vi "Add.vi"(7 "Top Level Library?":bool, 8 "error in (no error)":errorcluster, 10 "ProjectItem Refnum":refnum<vi>, 11 "PPL in":refnum<class "NI_AB_API_PPL.lvclass">) -> (0 "error out":errorcluster, 3 "PPL out":refnum<class "NI_AB_API_PPL.lvclass">)   [LabVIEW 2020, in "NI_AB_API_PPL.lvclass"]
uses:
  <vilib>/AppBuilder/AB_API/PPL/NI_AB_API_PPL.lvclass
  e:/builds/penguin/labview/branches/2020/dev/dist/vi.lib/AppBuilder/AB_API/Build/NI_AB_API_Build.lvclass
  <vilib>/AppBuilder/AB_Classes/PackedLib/AB_PackedLibrary.lvclass
  e:/builds/penguin/labview/branches/2020/dev/dist/vi.lib/AppBuilder/AB_Classes/Build/AB_Build.lvclass
  <vilib>/AppBuilder/AB_API/PPL/NI_AB_API_PPL.lvclass/NI_AB_API_PPL.ctl
  <vilib>/AppBuilder/AB_Classes/Build/AB_Build.lvclass
  <vilib>/AppBuilder/AB_Classes/Source/AB_Source.lvclass
  <vilib>/AppBuilder/AB_API/Build/NI_AB_API_Build.lvclass
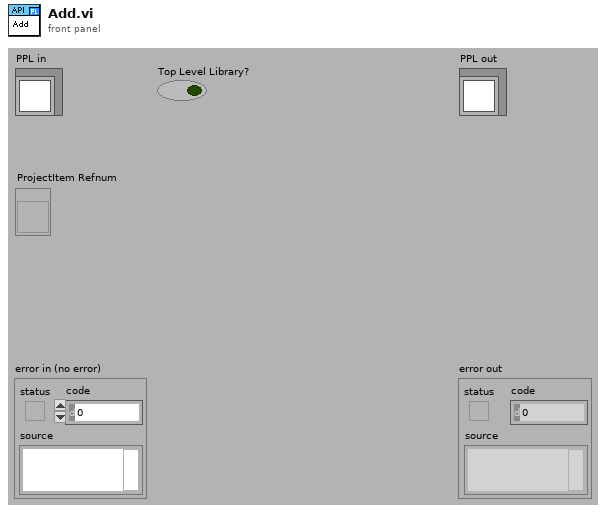
[diagram p1: front panel]
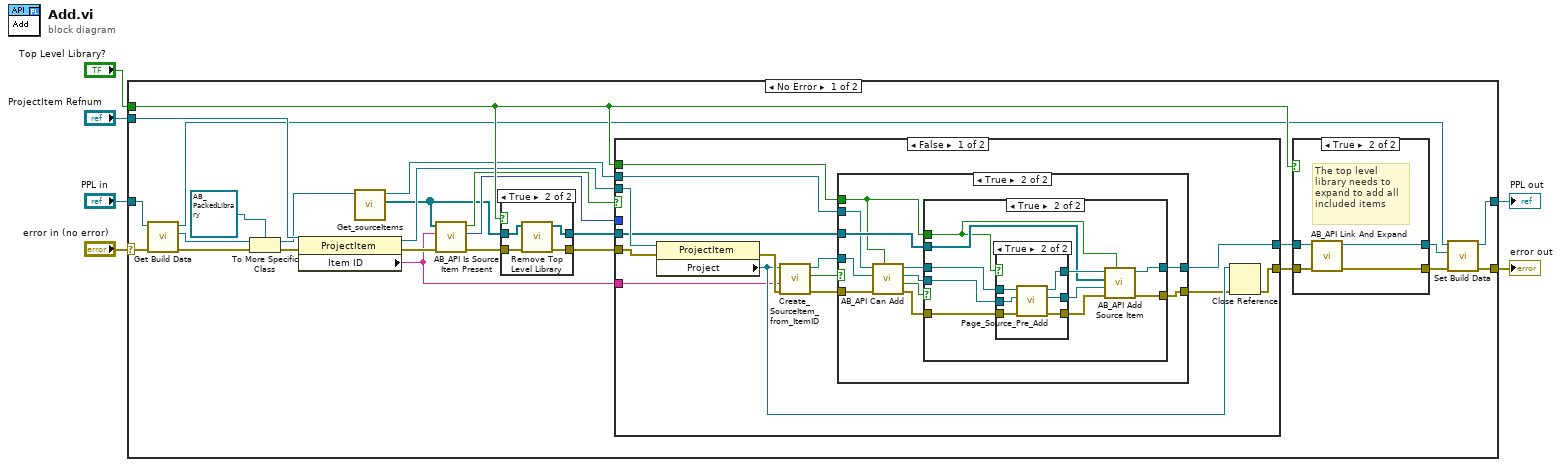
[diagram p0: block diagram]
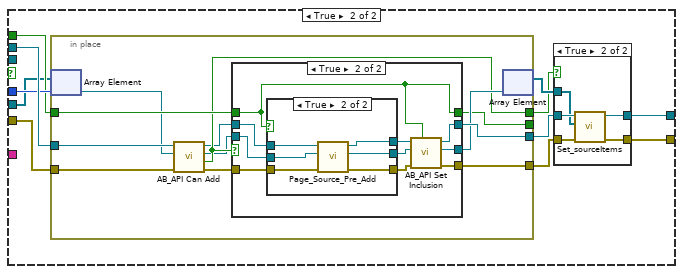
[diagram p7: hidden frame]
diagram:
  n1 = case shown="No Error" "error in (no error)" {
    selector: "error in (no error)" -> [w31 w147]
    tunnel: [w11 w147] -> w5
    tunnel: [w13 w146] -> w3
    tunnel: "PPL in" -> [w8 w146]
    tunnel: "ProjectItem Refnum" -> [w32 _]
    tunnel: "Top Level Library?" -> [w30 _]
    frame No Error {
      n2 = call <vilib>:"Get Build Data.vi"("error in (no error)"=w31, "NI_AB_API_Build in"=w8) -> ("error out"=w16:errorcluster, "AB_Build.lvclass"=w9:refnum<class "AB_Build.lvclass">, "NI_AB_API_Build out"=w7:refnum<class "NI_AB_API_PPL.lvclass">)  [unwired: 7 in]
      n3 = To More Specific Class(target class=refnum<class "AB_PackedLibrary.lvclass"> refnum ("AB_PackedLibrary.lvclass"), reference=w9, error in=w16) -> (specific class reference=w14:refnum<class "AB_PackedLibrary.lvclass">, error out=w15:errorcluster)
      n4 = property class="ProjectItem"(reference=w32, error in=w15) -> (reference out=w29:refnum<vi>, error out=w26:errorcluster, "Item ID"=w25:string)
      n5 = call <vilib>:"Get_sourceItems.vi"("Class in"=w14) -> ("sourceItems"=w23:refnum<class "AB_Source.lvclass">[], "Class out"=w28:refnum<class "AB_PackedLibrary.lvclass">)  [unwired: 8 in, 1 out]
      n6 = call <vilib>:"AB_API Is Source Item Present.vi"("error in"=w26, "item ID"=w25, "source items"=w23) -> ("error out"=w21:errorcluster, "index"=w24:i32, "source item present?"=w27:bool)  [unwired: 6 in]
      n7 = case shown="True" w30 {
        tunnel: w23 -> [w40 w44]
        tunnel: [w40 w43] -> w22
        tunnel: w21 -> [w39 w42]
        tunnel: [w39 w41] -> w20
        frame False {
        }
        frame True {
          n8 = call <vilib>:"Remove Top Level Library.vi"("error in"=w42, "sourceItems"=w44) -> ("error out"=w41:errorcluster, "sourceItems out"=w43:refnum<class "AB_Source.lvclass">[])  [unwired: 7 in]
        }
      }
      n9 = case shown="False" w27 {
        tunnel: w29 -> [w58 _]
        tunnel: [w54 w100] -> w19
        tunnel: [w50 w98] -> w18
        tunnel: w20 -> [w49 w94]
        tunnel: w28 -> [w48 w103]
        tunnel: w25 -> [w47 _]
        tunnel: w22 -> [w46 w95]
        tunnel: w24 -> [_ w102]
        tunnel: w30 -> [w45 w97]
        frame False {
          n10 = property class="ProjectItem"(reference=w58, error in=w49) -> (error out=w57:errorcluster, "Project"=w52:refnum<vi>)  [unwired: 1 out]
          n11 = call <vilib>:"Create_SourceItem_from_ItemID.vi"("error in (no error)"=w57, "itemID"=w47, "Project Refnum"=w52) -> ("error out"=w55:errorcluster, "valid?"=w53:bool, "AB_Source out"=w56:refnum<class "AB_Source.lvclass">)  [unwired: 6 in]
          n12 = case shown="True" w53 {
            tunnel: w56 -> [_ w68]
            tunnel: w55 -> [w59 w64]
            tunnel: w48 -> [w60 w67]
            tunnel: [w60 w71] -> w54
            tunnel: [w59 w70] -> w51
            tunnel: w46 -> [_ w69]
            tunnel: w45 -> [_ w61]
            frame False {
            }
            frame True {
              n13 = call <vilib>:"AB_API Can Add.vi"("top tree? (true)"=w61, "error in (no error)"=w64, "AB_Source in"=w68, "Build in"=w67) -> ("error out"=w63:errorcluster, "can add?"=w62:bool, "AB_Source out"=w65:refnum<class "AB_Source.lvclass">, "Build out"=w66:refnum<class "AB_PackedLibrary.lvclass">)  [unwired: 4 in]
              n14 = case shown="True" w62 {
                tunnel: w66 -> [w73 w81]
                tunnel: [w73 w82] -> w71
                tunnel: [w72 w83] -> w70
                tunnel: w63 -> [w72 w76]
                tunnel: w65 -> [_ w79]
                tunnel: w69 -> [_ w77]
                tunnel: w61 -> [_ w74]
                frame False {
                }
                frame True {
                  n15 = case shown="True" w74 {
                    tunnel: w81 -> [w86 w92]
                    tunnel: [w86 w91] -> w80
                    tunnel: w79 -> [w85 w90]
                    tunnel: [w85 w89] -> w78
                    tunnel: w76 -> [w84 w88]
                    tunnel: [w84 w87] -> w75
                    frame False {
                    }
                    frame True {
                      n16 = call-dynamic "Page_Source_Pre_Add.vi"("error in (no error)"=w88, "AB_Source in"=w90, "AB_PackedLibrary in"=w92) -> ("error out"=w87:errorcluster, "AB_Source out"=w89:refnum<class "AB_Source.lvclass">, "AB_PackedLibrary out"=w91:refnum<class "AB_PackedLibrary.lvclass">)  [unwired: 6 in]
                    }
                  }
                  n17 = call <vilib>:"AB_API Add Source Item.vi"("top tree? (true)"=w74, "error in"=w75, "Source in"=w78, "source items"=w77, "Build in"=w80) -> ("error out"=w83:errorcluster, "Build out"=w82:refnum<class "AB_PackedLibrary.lvclass">)  [unwired: 5 in]
                }
              }
            }
          }
          n18 = Close Reference(reference=w52, error in (no error)=w51) -> (error out=w50:errorcluster)
        }
        frame True {
          n19 = in-place {
            in-place-border: [w122] -> w101
            in-place-border: w103 -> [w117]
            in-place-border: w94 -> [w112]
            in-place-border: [w121] -> w99
            in-place-border: w97 -> [w119]
            in-place-border: [w118] -> w93
            in-place-border: [w111] -> _
            n20 = in-place-array #1(w95, w102) -> (w113:refnum<class "AB_Source.lvclass">)
            n21 = call <vilib>:"AB_API Can Add.vi"("error in (no error)"=w112, "AB_Source in"=w113, "Build in"=w117) -> ("error out"=w114:errorcluster, "can add?"=w118:bool, "AB_Source out"=w115:refnum<class "AB_Source.lvclass">, "Build out"=w116:refnum<class "AB_PackedLibrary.lvclass">)  [unwired: 5 in]
            n22 = case shown="True" w118 {
              tunnel: [w124 w134] -> w121
              tunnel: [w126 w136] -> w122
              tunnel: w116 -> [w126 w129]
              tunnel: w115 -> [w125 w133]
              tunnel: w114 -> [w124 w131]
              tunnel: [w125 w135] -> w120
              tunnel: w119 -> [w123 w127]
              tunnel: [w123 w127] -> w111
              frame False {
              }
              frame True {
                n23 = case shown="True" w127 {
                  tunnel: w133 -> [w139 w145]
                  tunnel: [w139 w144] -> w132
                  tunnel: w131 -> [w138 w141]
                  tunnel: [w138 w140] -> w130
                  tunnel: w129 -> [w137 w143]
                  tunnel: [w137 w142] -> w128
                  frame False {
                  }
                  frame True {
                    n24 = call-dynamic "Page_Source_Pre_Add.vi"("error in (no error)"=w141, "AB_Source in"=w145, "AB_PackedLibrary in"=w143) -> ("error out"=w140:errorcluster, "AB_Source out"=w144:refnum<class "AB_Source.lvclass">, "AB_PackedLibrary out"=w142:refnum<class "AB_PackedLibrary.lvclass">)  [unwired: 6 in]
                  }
                }
                n25 = call <vilib>:"AB_API Set Inclusion.vi"("top tree? (true)"=w127, "error in (no error)"=w130, "Source in"=w132, "Build in"=w128) -> ("error out"=w134:errorcluster, "AB_Source_VI out"=w135:refnum<class "AB_Source.lvclass">, "AB_Build out"=w136:refnum<class "AB_PackedLibrary.lvclass">)  [unwired: 5 in]
              }
            }
            n26 = in-place-array #1(w120) -> (w96:refnum<class "AB_Source.lvclass">[])  [unwired: 1 out]
          }
          n27 = case shown="True" w93 {
            tunnel: w101 -> [w105 w108]
            tunnel: [w105 w110] -> w100
            tunnel: w99 -> [w104 w106]
            tunnel: [w104 w109] -> w98
            tunnel: w96 -> [_ w107]
            frame False {
            }
            frame True {
              n28 = call <vilib>:"Set_sourceItems.vi"("error in (no error)"=w106, "sourceItems"=w107, "Class in"=w108) -> ("error out"=w109:errorcluster, "Class out"=w110:refnum<class "AB_PackedLibrary.lvclass">)  [unwired: 7 out]
            }
          }
        }
      }
      n29 = case shown="True" w30 {
        tunnel: w19 -> [w34 w38]
        tunnel: [w34 w37] -> w12
        tunnel: w18 -> [w33 w36]
        tunnel: [w33 w35] -> w10
        frame False {
        }
        frame True {
          # "The top level\nlibrary needs to \nexpand to add all \nincluded items"
          n30 = call <vilib>:"AB_API Link And Expand.vi"("error in"=w36, "Build in"=w38) -> ("error out"=w35:errorcluster, "Build out"=w37:refnum<class "AB_PackedLibrary.lvclass">)  [unwired: 8 in]
        }
      }
      n31 = call <vilib>:"Set Build Data.vi"("error in (no error)"=w10, "AB_Build.lvclass"=w12, "NI_AB_API_Build in"=w7) -> ("error out"=w11:errorcluster, "NI_AB_API_Build out"=w13:refnum<class "NI_AB_API_PPL.lvclass">)  [unwired: 7 in]
    }
    frame Error {
    }
  }
  "error out" <- w5
  "PPL out" <- w3
